vi "Pre Launch Init.vi"(11 "ConnectionReader in":refnum<class "ConnectionReader.lvclass">) -> (0 "error out":errorcluster, 3 "ConnectionReader out":refnum<class "ConnectionReader.lvclass">)   [LabVIEW 2019, in "ConnectionReader.lvlib" / "ConnectionReader.lvclass"]
doc: "(<B>Filename</B>: Actor Framework.lvlib:Actor.lvclass:Pre Launch Init.vi)\n\nDefines behavior that occurs after the Launch Nested Actor method is invoked but before the actor's Actor Core method begins running.\n\nBy default, this method does nothing. A descendant class may override it to define behavior."
uses:
  <vilib>/gpm_packages/@cs/Network-interface/Source/ConnectionReader/ConnectionReader/ConnectionReader.lvclass
  C:/Program Files/National Instruments/LabVIEW 2019/vi.lib/ActorFramework/Actor/Actor.lvclass
  <vilib>/ActorFramework/Actor/Actor.lvclass/Actor.ctl
  <vilib>/ActorFramework/Message Enqueuer/Message Enqueuer.lvclass/Message Enqueuer.ctl
  <vilib>/ActorFramework/Message Enqueuer/Init from Existing Queue.vi
  <vilib>/ActorFramework/Message Enqueuer/Enqueue.vi
  <vilib>/gpm_packages/@cs/Network-interface/Source/ConnectionReader/ConnectionReader Messages/Wait on Message Msg/Wait on Message Msg.lvclass
  C:/Program Files/National Instruments/LabVIEW 2019/vi.lib/ActorFramework/Message/Message.lvclass
  <vilib>/ActorFramework/Message Priority Queue/Priority Enqueue.vi
  <vilib>/gpm_packages/@cs/Network-interface/Source/Logged Actor/LoggedActor.lvclass
  <vilib>/ActorFramework/Message Enqueuer/Message Enqueuer.lvclass
  <vilib>/ActorFramework/Actor/Actor.lvclass
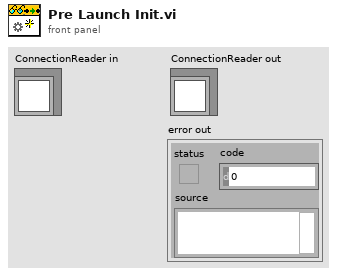
[diagram p1: front panel]
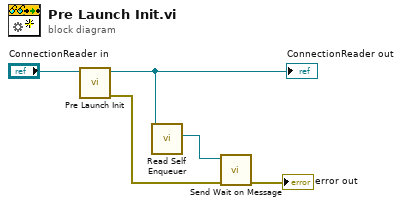
[diagram p0: block diagram]
diagram:
  n1 = call-parent "Pre Launch Init.vi"("Logged Actor in"="ConnectionReader in") -> ("error out"=w2:errorcluster, "Logged Actor out"=w4:refnum<class "ConnectionReader.lvclass">)  [unwired: 9 in]
  "ConnectionReader out" <- w4
  n2 = call <vilib>:"Read Self Enqueuer.vi"("Actor"=w4) -> ("Self Enqueuer"=w3:refnum<class "Message Enqueuer.lvclass">)  [unwired: 10 in]
  n3 = call <vilib>:"Send Wait on Message.vi"("error in (no error)"=w2, "Message Enqueuer"=w3) -> ("error out"=→"error out":errorcluster)  [unwired: 8 in, 1 out]
